vi "pH_val.vi"() -> (3 "return value":dbl)   [LabVIEW 2024]
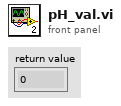
[diagram p1: front panel]
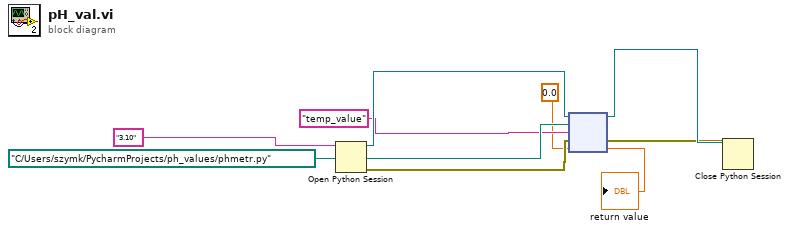
[diagram p0: block diagram]
diagram:
  n1 = Open Python Session(python version="3.10" ("Python version")) -> (session out=w7:refnum<k35>, error out=w4:errorcluster)  [unwired: 2 in]
  n2 = node(w7, path "C:/Users/szymk/PycharmProjects/ph_values/phmetr.py" ("module path"), "temp_value", w4, 0.0) -> (w2:refnum<k35>, w1:errorcluster, →"return value":dbl)  [unwired: 2 out]
  n3 = Close Python Session(session in=w2, error in=w1) -> ()  [unwired: 1 out]
